vi "uActor_Set_uErrClass(Superseding).vi"(10 "uErr":refnum<class "uErr.lvclass">, 11 "uActor in":refnum<class "uActor.lvclass">) -> (3 "uActor out":refnum<class "uActor.lvclass">)   [LabVIEW 2023, in "uLib.lvlib" / "uActor.lvclass"]
doc: "Use at runtime to set the Error handling behavior of an actor. Invoking this method overrides any previously assigned uError class."
uses:
  uActor.lvclass
  uErr/uErr/uErr.lvclass
  uActor.lvclass/uActor.ctl
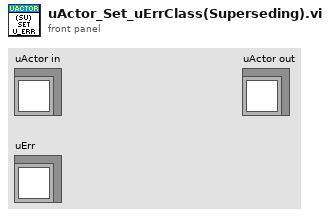
[diagram p1: front panel]
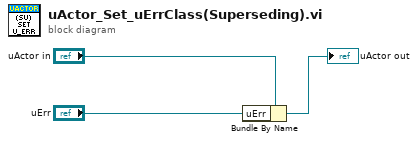
[diagram p0: block diagram]
diagram:
  n1 = Bundle By Name(cluster="uActor in", "uErr"="uErr") -> (→"uActor out":refnum<class "uActor.lvclass">)
